vi "Cluster Ref to Strings.vi"(0 "control ref":refnum<vi>, 11 "error in (no error)":errorcluster) -> (4 "Strings[]":string[](array[string]), 15 "error out":errorcluster)   [LabVIEW 2020]
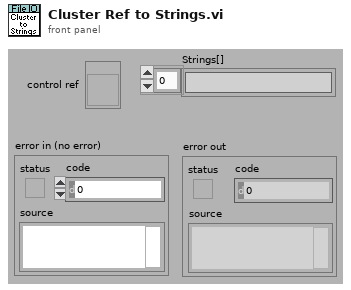
[diagram p1: front panel]
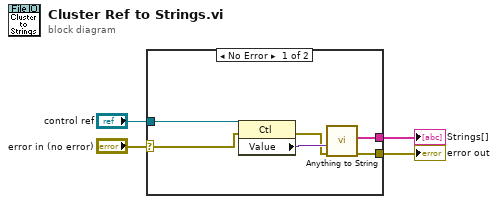
[diagram p0: block diagram]
diagram:
  n1 = case shown="No Error" "error in (no error)" {
    selector: "error in (no error)" -> [w5 w11]
    tunnel: "control ref" -> [w6 _]
    tunnel: [w8 _] -> w4
    tunnel: [w7 w11] -> w2
    frame No Error {
      n2 = property class="Ctl"(reference=w6, error in=w5) -> (error out=w9:errorcluster, "Value"=w10:variant)  [unwired: 1 out]
      n3 = call "Anything to String.vi"("Error In"=w9, "Anything"=w10) -> ("Error Out"=w7:errorcluster, "Strings[]"=w8:string[])  [unwired: 7 in, 1 out]
    }
    frame Error {
    }
  }
  "error out" <- w2
  "Strings[]" <- w4
